vi "umTomm.vi"(1 "distance (um)":dbl) -> (0 "distance (mm)":dbl)   [LabVIEW 2015]
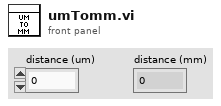
[diagram p1: front panel]
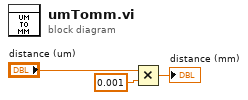
[diagram p0: block diagram]
diagram:
  n1 = Multiply(x="distance (um)", y=0.001) -> (x*y=→"distance (mm)":dbl)
